vi "Example.vi"() -> ()   [LabVIEW 2019, in "MicronTemplateAPIs.lvlib" / "MicronTemplateAPIs.lvclass"]
uses:
  MicronTemplateAPIs.lvclass
  Base/Client/Typedefs/Service Details.ctl
  Base/Client/MicronClient.lvclass
  gRPC/Client/MicronGRPCClient.lvclass
  <vilib>/SLL Toolkit/SLL File IO/SLL File IO.lvlib
panel:
  in  "Connection Type":enum32{"Start New", "Connect Existing"}(tab)=enum."Connect Existing"
  in  "Path":path=path "../Builds/GRPC/Server/GRPCServerExample.exe"
  in  "Port":i32=50051
  in  "Connection String":string="localhost:50051"
  out "error out":errorcluster
  out "Response":string
  in  "Command":string="Hello World!"
  in  "Payload":string="Popping in to say hi!"
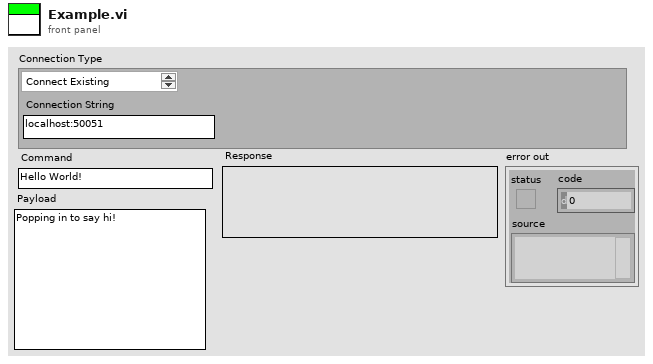
[diagram p1: front panel]
types:
  T1 = typedef "MicronClient.lvclass/Service Details.ctl" = cluster{"Micron Path":path, "Network":string, "Name":string, "Port":i32, "Args":string}
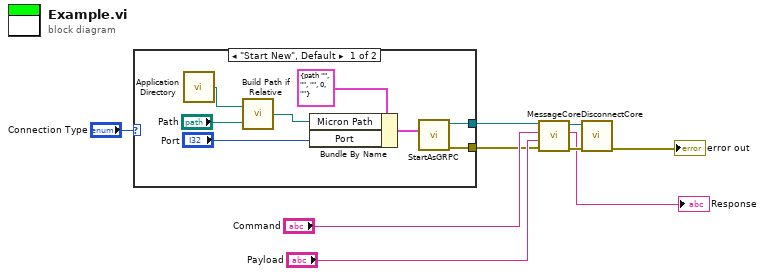
[diagram p0: block diagram]
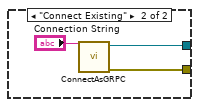
[diagram p2: hidden frame]
diagram:
  n1 = case shown="\"Start New\", Default" "Connection Type" {
    tunnel: [w17 w20] -> w2
    tunnel: [w16 w19] -> w1
    frame "Start New", Default {
      n2 = call <vilib>:"Application Directory.vi"() -> ("Application Directory"=w10:path)
      n3 = call <vilib>:"Build Path if Relative.vi"("Relative or Absolute Path"="Path", "Base Path"=w10) -> ("Path Out"=w11:path)
      n4 = Bundle By Name(cluster=T1 {"Micron Path"=path "", "Network"="", "Name"="", "Port"=0, "Args"=""} ("Service Details"), "Micron Path"=w11, "Port"="Port") -> (w14:T1)
      n5 = call "StartAsGRPC.vi"("Service Details"=w14) -> ("error out"=w17:errorcluster, "MicronClient out"=w16:refnum<class "MicronClient.lvclass">)  [unwired: 9 in]
    }
    frame "Connect Existing" {
      n6 = call "ConnectAsGRPC.vi"("Connection String"="Connection String") -> ("error out"=w20:errorcluster, "MicronClient out"=w19:refnum<class "MicronClient.lvclass">)  [unwired: 9 in]
    }
  }
  n7 = call-dynamic "MessageCore.vi"("error in (no error)"=w2, "Payload"="Payload", "Command"="Command", "MicronClient in"=w1) -> ("error out"=w8:errorcluster, "Response"=→"Response":string, "MicronClient out"=w9:refnum<class "MicronClient.lvclass">)  [unwired: 5 in]
  n8 = call-dynamic "DisconnectCore.vi"("error in (no error)"=w8, "MicronClient in"=w9) -> ("error out"=→"error out":errorcluster)  [unwired: 8 in, 1 out]
